vi "svl_Exp Avg Resampled Level (N Ch).vi"(5 "timeConstant":dbl=1.0 format="%.3f", 7 "exponential mode":enum16{"Slow", "Fast", "Impulse", "Custom"}(ring)=enum."Fast", 8 "error in (no error)":errorcluster, 9 "processing state":T1(ring), 11 "scaled signals":T2(array[cluster]) {"even angle signal" format="%.2f"; "dr" format="%.2f"; "r0" format="%.2f"}) -> (0 "error out":errorcluster, 1 "dup processing state":T1(ring), 3 "exp avg signals":T2(array[cluster]) {"even angle signal" format="%.2f"; "dr" format="%.2f"; "r0" format="%.2f"}, 4 "actual time constant [ms]":dbl=125.0 format="%.2f")   [LabVIEW 2017]
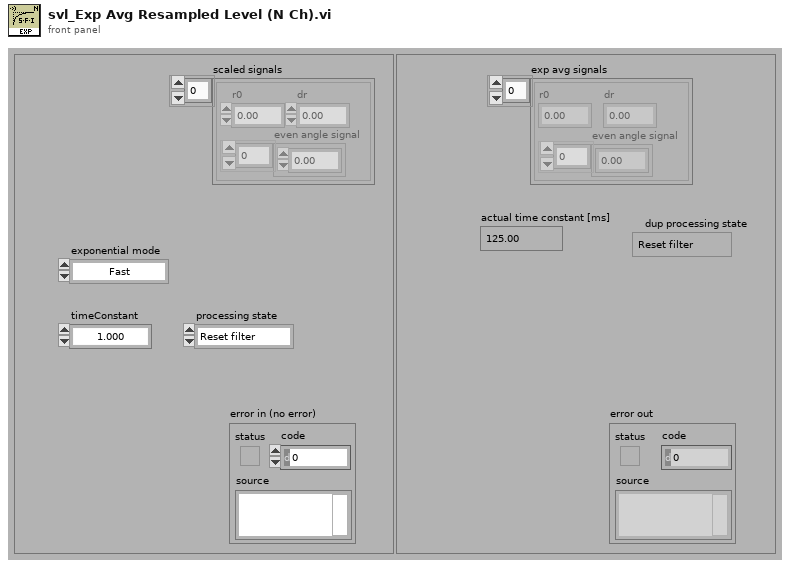
[diagram p1: front panel]
types:
  T1 = enum16{"Reset filter", "Restart averaging", "Continue processing"}
  T2 = cluster{"r0":dbl, "dr":dbl, "even angle signal":dbl[]}[]
  T3 = cluster{"Reverse Coefficients":dbl[], "Forward Coefficients":dbl[]}
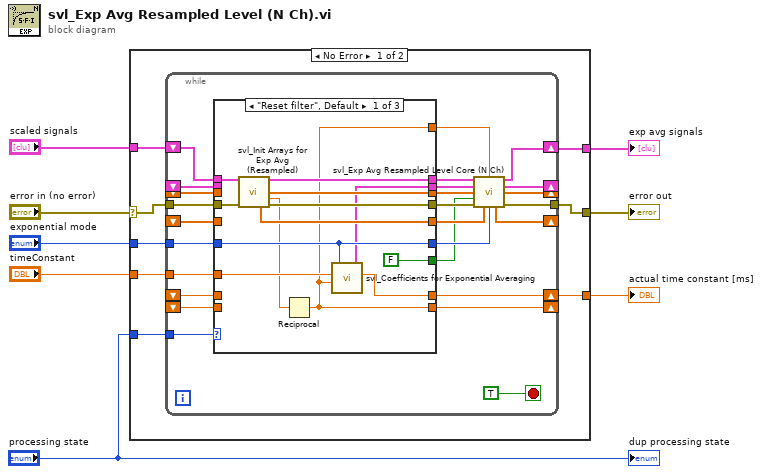
[diagram p0: block diagram]
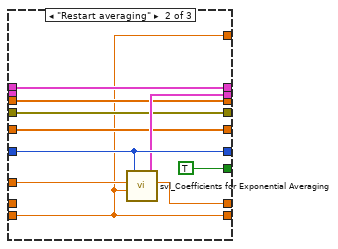
[diagram p2: hidden frame]
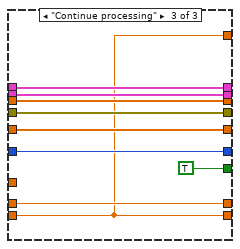
[diagram p3: hidden frame]
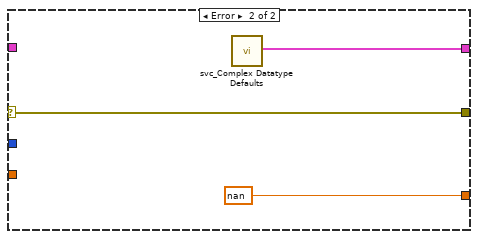
[diagram p4: hidden frame]
diagram:
  n1 = case shown="No Error" "error in (no error)" {
    selector: "error in (no error)" -> [w14 w77]
    tunnel: "processing state" -> [w16 _]
    tunnel: "scaled signals" -> [w15 _]
    tunnel: "exponential mode" -> [w13 _]
    tunnel: "timeConstant" -> [w12 _]
    tunnel: [w11 w77] -> w3
    tunnel: [w10 nan ("actual time constant [ms]")] -> w2
    tunnel: [w9 w75] -> w1
    frame No Error {
      n2 = while {
        shift-left: _ -> [w30]
        shift-right: [w24] -> _
        shift-left: _ -> [w31]
        shift-right: [w32] -> w10
        tunnel: [w23] -> w11
        shift-left: _ -> [w33]
        shift-right: [w26] -> _
        shift-left: _ -> [w35]
        shift-right: [w36] -> _
        shift-left: _ -> [w34]
        shift-right: [w20] -> _
        tunnel: w12 -> [w37]
        tunnel: w13 -> [w38]
        tunnel: w14 -> [w39]
        tunnel: w16 -> [w42]
        shift-right: [w17] -> w9
        shift-left: w15 -> [w40]
        stop <- TRUE stop-if-true
        n3 = case shown="\"Reset filter\", Default" w42 {
          tunnel: w40 -> [w55 w62 w71]
          tunnel: w39 -> [w54 w58 w69]
          tunnel: w38 -> [w51 w61 w72]
          tunnel: w37 -> [w53 w65 _]
          tunnel: [w44 w56 w66] -> w36
          tunnel: w35 -> [_ w56 w66]
          tunnel: w34 -> [_ _ w67]
          tunnel: [w46 w57 w68] -> w27
          tunnel: w33 -> [_ w57 w68]
          tunnel: [w47 w58 w69] -> w28
          tunnel: [w52 w64 w74] -> w32
          tunnel: w31 -> [_ _ w74]
          tunnel: [w48 w59 w70] -> w29
          tunnel: w30 -> [_ w59 w70]
          tunnel: [w51 w61 w72] -> w25
          tunnel: [w45 w60 w67] -> w19
          tunnel: [FALSE ("init/cont (init:F)") TRUE ("init/cont (init:F)") TRUE ("init/cont (init:F)")] -> w22
          tunnel: [w49 w62 w71] -> w21
          tunnel: [w44 w56 w66] -> w18
          frame "Reset filter", Default {
            n4 = call <vilib>:"svl_Init Arrays for Exp Avg (Resampled).vi"("scaled signals"=w55, "error in (no error)"=w54) -> ("scaled signals"=w49:T2, "initial values (impulse)"=w48:dbl[], "dr"=w43:dbl, "initial values (exp)"=w46:dbl[], "error out"=w47:errorcluster)  [unwired: 9 in]
            n5 = Reciprocal(x=w43) -> (1/x=w44:dbl)
            n6 = call <vilib>:"svl_Coefficients for Exponential Averaging.vi"("sampling frequency [Hz]"=w44, "time constant [ms]"=w53, "exponential mode"=w51) -> ("actual time constant [ms]"=w52:dbl, "filter coefficients"=w45:T3)  [unwired: 3 in]
          }
          frame "Restart averaging" {
            n7 = call <vilib>:"svl_Coefficients for Exponential Averaging.vi"("sampling frequency [Hz]"=w56, "time constant [ms]"=w65, "exponential mode"=w61) -> ("actual time constant [ms]"=w64:dbl, "filter coefficients"=w60:T3)  [unwired: 3 in]
          }
          frame "Continue processing" {
          }
        }
        n8 = call <vilib>:"svl_Exp Avg Resampled Level Core (N Ch).vi"("scaled signals"=w21, "sampling frequency [Hz]"=w18, "filter coefficients (in)"=w19, "initial values (impulse)"=w29, "init/cont (init:F)"=w22, "error in (no error)"=w28, "initial values (exp)"=w27, "exponential mode"=w25) -> ("exp avg signals"=w17:T2, "dup filter coefficients"=w20:T3, "final values (impulse)"=w24:dbl[], "final values (exp)"=w26:dbl[], "error out"=w23:errorcluster)  [unwired: 3 in]
      }
    }
    frame Error {
      n9 = call <vilib>:"svc_Complex Datatype Defaults.vi"() -> ("empty array of spectra"=w75:cluster{"f0":dbl, "df":dbl, "magnitude":dbl[]}[])  [unwired: 11 in, 8 out]
    }
  }
  "exp avg signals" <- w1
  "error out" <- w3
  "actual time constant [ms]" <- w2
  "dup processing state" <- "processing state"
